vi "DrawARectangle.vi"(1 "height":i32, 2 "width":i32, 3 "y":i32, 4 "x":i32) -> (0 "picture":picture)   [LabVIEW 2010]
uses:
  <vilib>/Utility/miscctls.llb/LVBoundsTypeDef.ctl
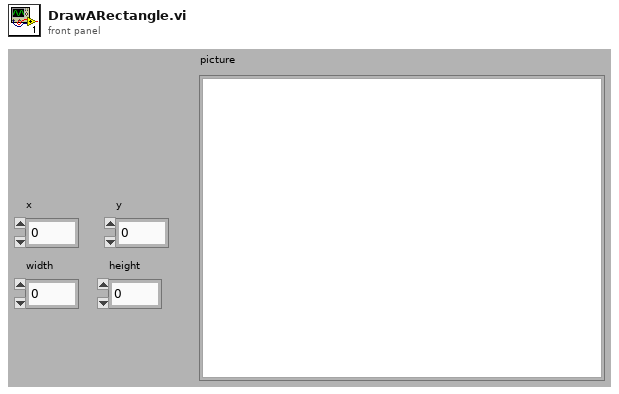
[diagram p1: front panel]
types:
  T1 = typedef "LVBoundsTypeDef.ctl" = cluster{"Width":u32, "Height":u32}
  T2 = cluster{"left":i16, "top":i16, "right":i16, "bottom":i16}
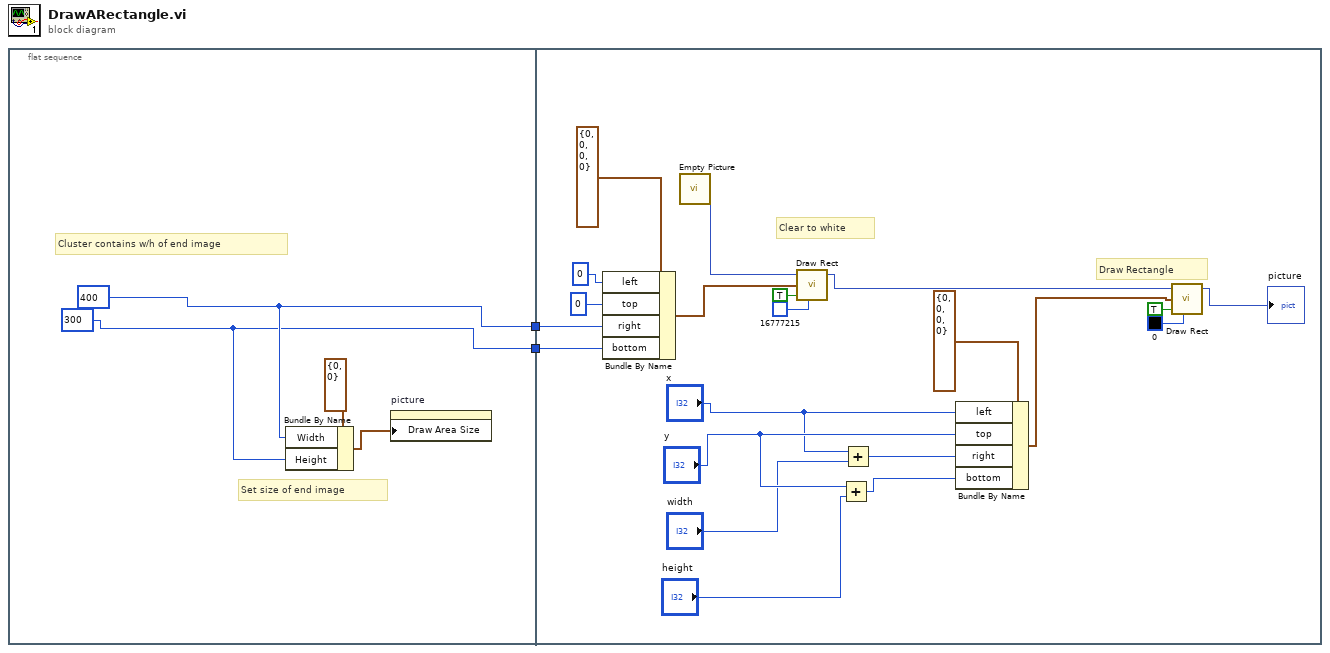
[diagram p0: block diagram]
diagram:
  n1 = flat-sequence {
    tunnel: [w4] -> w2
    tunnel: [w3] -> w1
    tunnel: w2 -> [w9]
    tunnel: w1 -> [w8]
    frame #0 {
      w3 = 300
      w4 = 400
      # "Set size of end image"
      # "Cluster contains w/h of end image"
      n2 = Bundle By Name(cluster=T1 {"Width"=0, "Height"=0} ("Draw Area Size"), "Width"=w4, "Height"=w3) -> (w5:T1)
      n3 = property on="picture" class="Pict"("Draw Area Size"=w5) -> ()  [unwired: 2 in, 2 out]
    }
    frame #1 {
      # "Draw Rectangle"
      # "Clear to white"
      n4 = Bundle By Name(cluster=T2 {"left"=0, "top"=0, "right"=0, "bottom"=0} ("rect"), "left"=0, "top"=0, "right"=w9, "bottom"=w8) -> (w16:T2)
      n5 = call "Empty Picture"() -> ("empty picture"=w7:picture)
      n6 = call <vilib>:"Draw Rect.vi"("picture"=w7, "rect"=w16, "fill?(F)"=TRUE, "color(black)"=u32 16777215) -> ("new picture"=w17:picture)  [unwired: 5 in]
      n7 = Add(x="y", y="height") -> (x+y=w22:i32)
      n8 = Add(x="x", y="width") -> (x+y=w21:i32)
      n9 = Bundle By Name(cluster=T2 {"left"=0, "top"=0, "right"=0, "bottom"=0} ("rect"), "left"="x", "top"="y", "right"=w21, "bottom"=w22) -> (w23:T2)
      n10 = call <vilib>:"Draw Rect.vi"("picture"=w17, "rect"=w23, "fill?(F)"=TRUE, "color(black)"=u32 0) -> ("new picture"=→"picture":picture)  [unwired: 5 in]
    }
  }
